vi "Master Setup Backup Scheduler.vi"(11 "Backup Path":path) -> ()   [LabVIEW 2017]
uses:
  Master Setup Backup Scheduler States.ctl
  <vilib>/Utility/config.llb/Read Key (Double).vi
  <vilib>/Utility/config.llb/Read Key (Boolean).vi
  <vilib>/Utility/config.llb/Read Key (U32).vi
  <vilib>/Utility/config.llb/Write Key (Double).vi
  <vilib>/Platform/browser.llb/Open URL in Default Browser (path).vi
  <vilib>/Utility/config.llb/Write Key (Boolean).vi
  <vilib>/Utility/config.llb/Write Key (U32).vi
  <vilib>/Utility/config.llb/NI_LVConfig.lvlib
panel:
  in  "Open Backup Directory":bool
  in  "Time Increment":enum32{"Days", "Weeks"}(ring)
  in  "Cancel":bool
  in  "Save":bool
  in  "Begin backup time":timestamp format="%<%b %d, %Y %I:%M %p>T"
  in  "Backup frequency":dbl
  out "Next scheduled backup":timestamp format="%<%b %d, %Y\n%I:%M %p>T"
  out "Last scheduled backup":timestamp format="%<%b %d, %Y\n%I:%M %p>T"
  in  "Auto Backup Enabled?":bool
  # "Back up the master setup files every"
  # "beginning on"
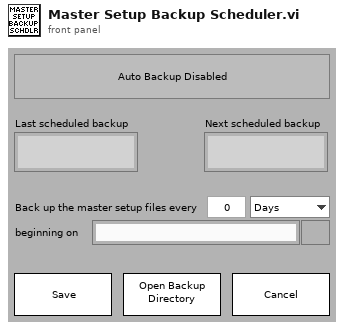
[diagram p1: front panel]
types:
  T1 = cluster{"Auto Backup Enabled?":bool, "Backup frequency":dbl, "Time Increment":enum32{"Days", "Weeks"}}
  T2 = typedef "Master Setup Backup Scheduler States.ctl" = enum16{"Initialize", "Enable/Disable controls", "Refresh controls", "Check for valid schdule", "Save", "Cancel", "Update", "Close", "Send backup command", "Update backup schedule", "Exit"}
  T3 = enum8{"Enabled", "Disabled", "Disabled and Grayed Out"}
  T4 = typedef "NI_LVConfig.lvlib/Config Data RefNum.ctl" = refnum<k1>
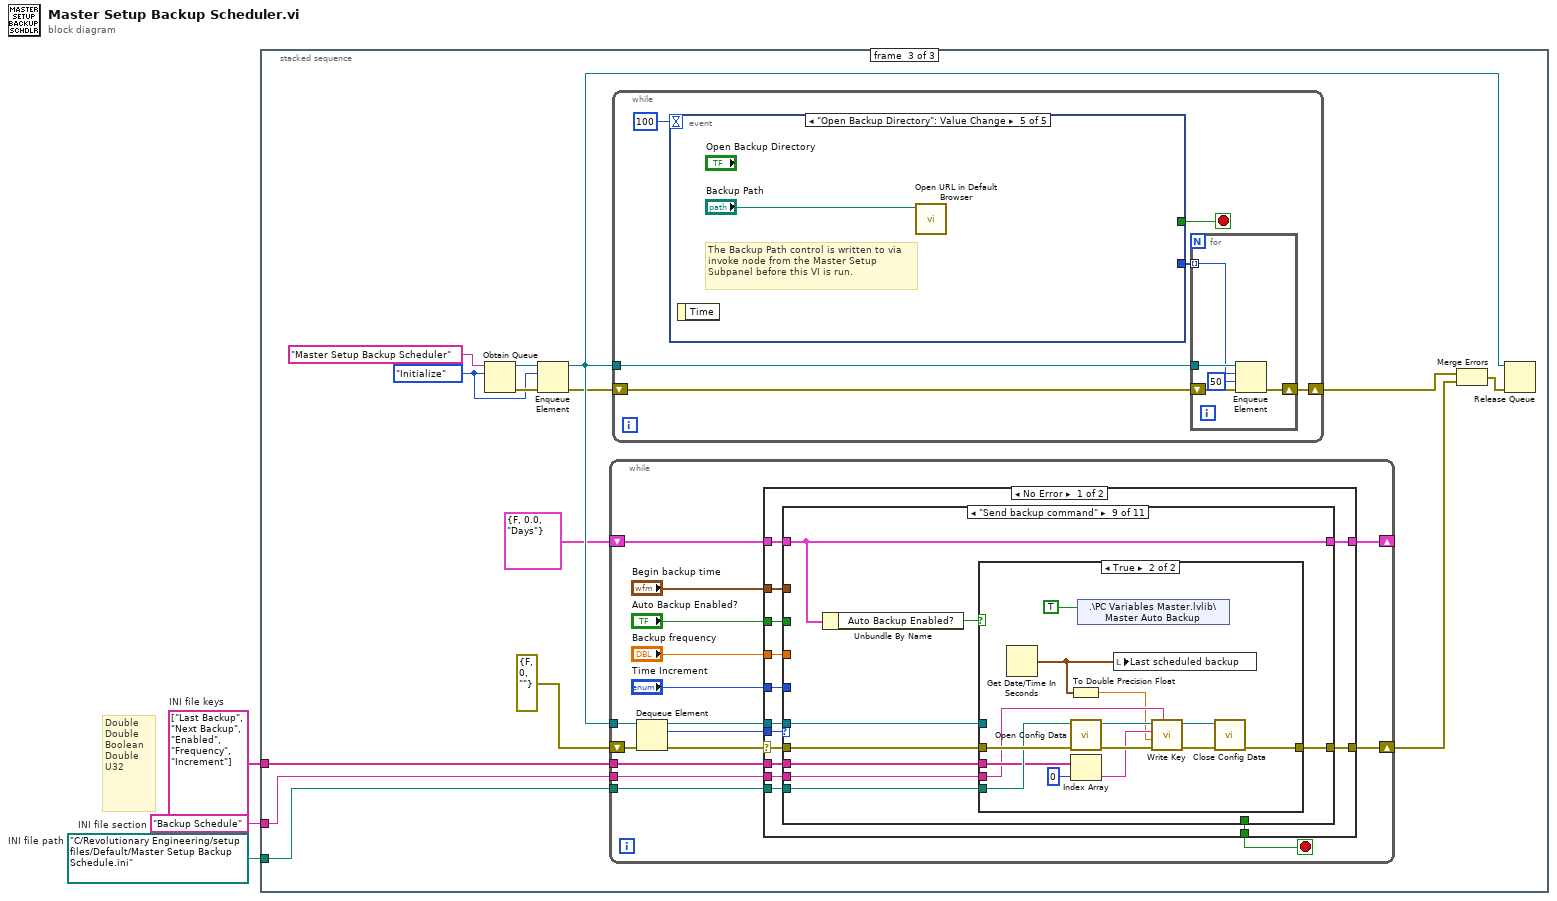
[diagram p0: block diagram]
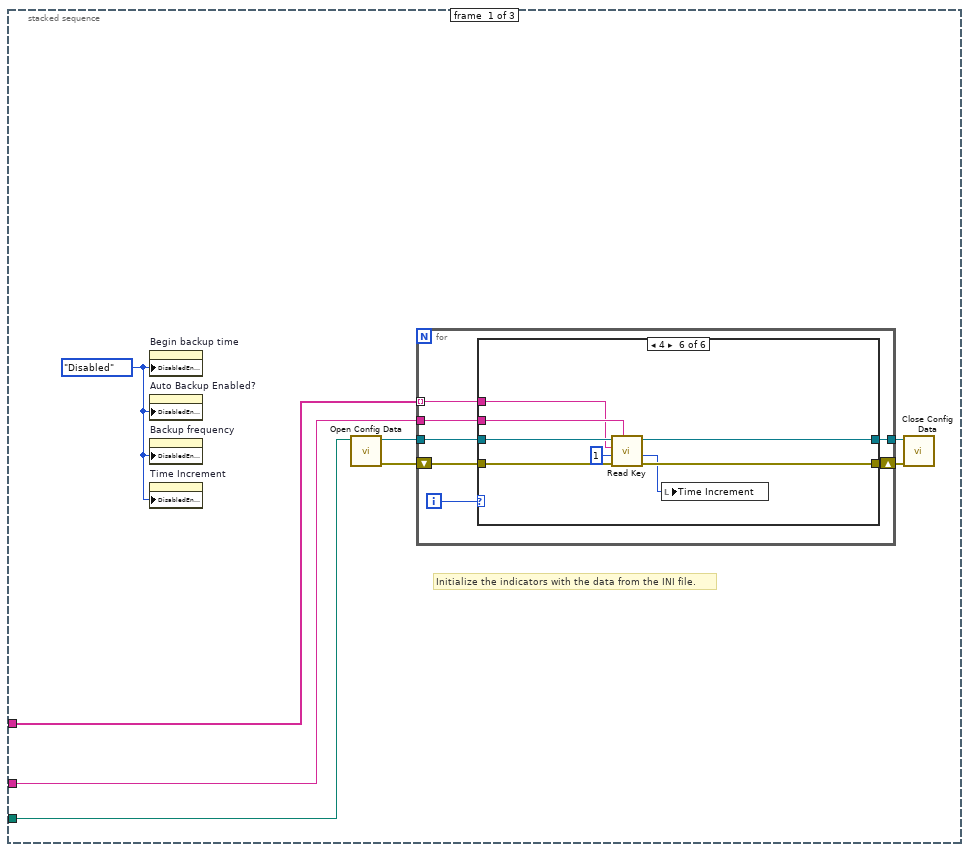
[diagram p2: hidden frame]
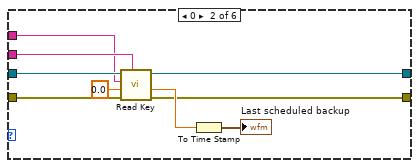
[diagram p4: hidden frame]
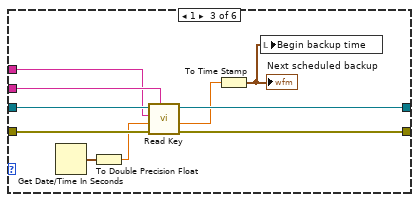
[diagram p5: hidden frame]
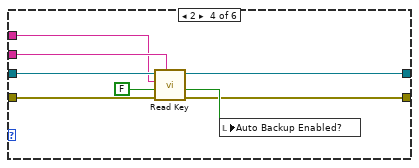
[diagram p6: hidden frame]
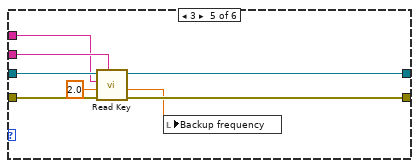
[diagram p7: hidden frame]
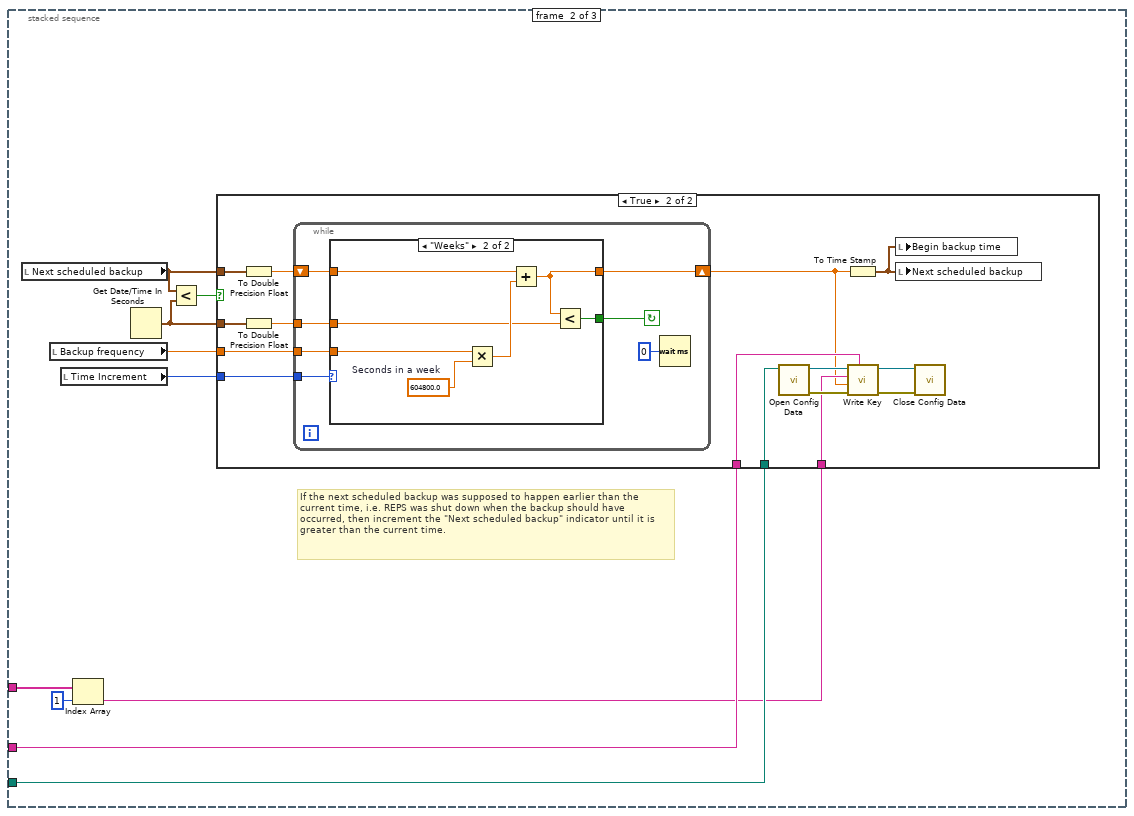
[diagram p8: hidden frame]
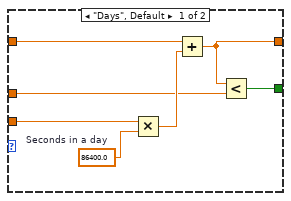
[diagram p10: hidden frame]
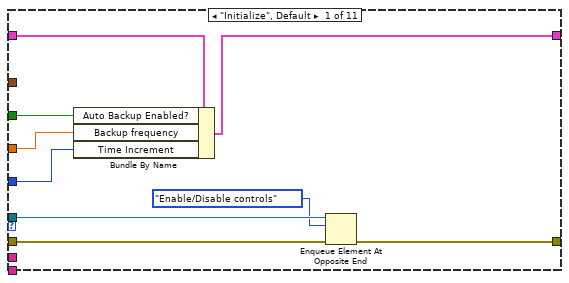
[diagram p11: hidden frame]
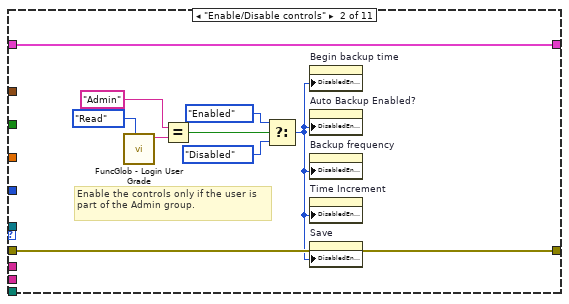
[diagram p12: hidden frame]
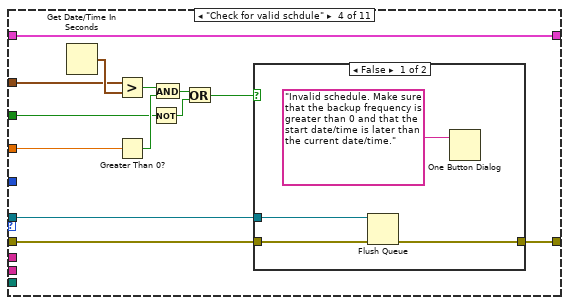
[diagram p14: hidden frame]
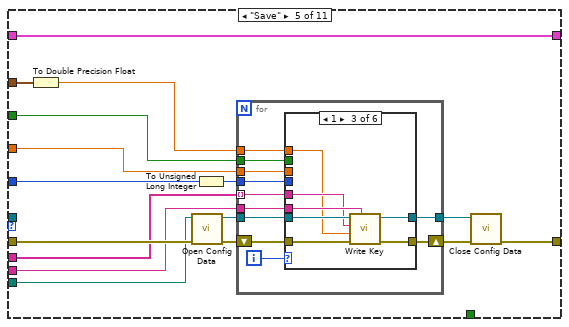
[diagram p16: hidden frame]
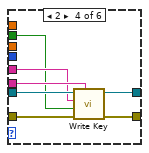
[diagram p19: hidden frame]
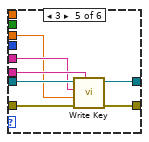
[diagram p20: hidden frame]
diagram:
  w1 = string[] ["Last Backup", "Next Backup", "Enabled", "Frequency", "Increment"]  # INI file keys
  w2 = "Backup Schedule"  # INI file section
  w3 = path "C:/Revolutionary Engineering/setup files/Default/Master Setup Backup Schedule.ini"  # INI file path
  # "Double\nDouble\nBoolean\nDouble\nU32"
  n1 = stacked-sequence {
    tunnel: w3 -> [w6 w68 w110]
    tunnel: w2 -> [w5 w67 w111]
    tunnel: w1 -> [w4 w66 w112]
    frame #0 {
      w7 = T3."Disabled" ("Disabled")
      # "Initialize the indicators with the data from the INI file."
      n2 = property on="Begin backup time" class="AbsTime (strict)"("DisabledEnum"=w7) -> ()  [unwired: 2 in, 2 out]
      n3 = property on="Auto Backup Enabled?" class="Bool (strict)"("DisabledEnum"=w7) -> ()  [unwired: 2 in, 2 out]
      n4 = property on="Backup frequency" class="DigNum (strict)"("DisabledEnum"=w7) -> ()  [unwired: 2 in, 2 out]
      n5 = property on="Time Increment" class="Enum (strict)"("DisabledEnum"=w7) -> ()  [unwired: 2 in, 2 out]
      n6 = call <vilib>:"Open Config Data.vi"("configuration file path"=w6) -> ("error out"=w10:errorcluster, "refnum"=w11:T4)  [unwired: 8 in, 1 out]
      n7 = for {
        tunnel: w11 -> [w17]
        tunnel: w5 -> [w14]
        tunnel: w4 -> [w15] mode=indexing
        shift-right: [w13] -> w9
        shift-left: w10 -> [w16]
        tunnel: [w12] -> w8
        i -> [w18]
        n8 = case shown="4" w18 {
          tunnel: w17 -> [w20 w29 w37 w47 w55 w63]
          tunnel: w16 -> [w19 w28 w39 w46 w54 w62]
          tunnel: w15 -> [_ w26 w34 w44 w52 w60]
          tunnel: w14 -> [_ w27 w35 w45 w53 w61]
          tunnel: [w19 w23 w38 w42 w50 w59] -> w13
          tunnel: [w20 w22 w36 w41 w51 w58] -> w12
          frame -1, Default {
          }
          frame 0 {
            n9 = call-poly <vilib>:"Read Key.vi"("section"=w27, "error in (no error)"=w28, "default value"=0.0, "key"=w26, "refnum"=w29) -> ("error out"=w23:errorcluster, "value"=w25:dbl, "refnum out"=w22:T4)  [unwired: 3 in, 1 out]
            n10 = To Time Stamp(1:w25) -> (0:→"Last scheduled backup":timestamp)
          }
          frame 1 {
            n11 = Get Date/Time In Seconds() -> (seconds since 1Jan1904=w32:timestamp)
            n12 = To Double Precision Float(number=w32) -> (double precision float=w31:dbl)
            n13 = call-poly <vilib>:"Read Key.vi"("section"=w35, "error in (no error)"=w39, "default value"=w31, "key"=w34, "refnum"=w37) -> ("error out"=w38:errorcluster, "value"=w33:dbl, "refnum out"=w36:T4)  [unwired: 3 in, 1 out]
            n14 = To Time Stamp(1:w33) -> (0:w30:timestamp)
            "Next scheduled backup" <- w30
            n15 = local write "Begin backup time"(w30) -> ()
          }
          frame 2 {
            n16 = call-poly <vilib>:"Read Key.vi"("section"=w45, "error in (no error)"=w46, "default value"=FALSE, "key"=w44, "refnum"=w47) -> ("error out"=w42:errorcluster, "value"=w43:bool, "refnum out"=w41:T4)  [unwired: 3 in, 1 out]
            n17 = local write "Auto Backup Enabled?"(w43) -> ()
          }
          frame 3 {
            n18 = call-poly <vilib>:"Read Key.vi"("section"=w53, "error in (no error)"=w54, "default value"=2.0, "key"=w52, "refnum"=w55) -> ("error out"=w50:errorcluster, "value"=w49:dbl, "refnum out"=w51:T4)  [unwired: 3 in, 1 out]
            n19 = local write "Backup frequency"(w49) -> ()
          }
          frame 4 {
            n20 = call-poly <vilib>:"Read Key.vi"("section"=w61, "error in (no error)"=w62, "default value"=u32 1, "key"=w60, "refnum"=w63) -> ("error out"=w59:errorcluster, "value"=w57:u32, "refnum out"=w58:T4)  [unwired: 3 in, 1 out]
            n21 = local write "Time Increment"(w57) -> ()
          }
        }
      }
      n22 = call <vilib>:"Close Config Data.vi"("error in (no error)"=w9, "refnum"=w8) -> ()  [unwired: 8 in, 2 out]
    }
    frame #1 {
      # "If the next scheduled backup was supposed to happen earlier than the current time, i.e. REPS was shut down when the backup should have occurred, then increment the \"Next scheduled backup\" indicator until it is greater than the current time."
      n23 = local read "Next scheduled backup"() -> (w70:timestamp)
      n24 = local read "Backup frequency"() -> (w72:dbl)
      n25 = local read "Time Increment"() -> (w71:enum32{"Days", "Weeks"})
      n26 = Index Array(array=w66, index=1) -> (element=w64:string)
      n27 = Get Date/Time In Seconds() -> (seconds since 1Jan1904=w69:timestamp)
      n28 = Less?(x=w70, y=w69) -> (x < y?=w73:bool)
      n29 = case shown="True" w73 {
        tunnel: w72 -> [_ w87]
        tunnel: w71 -> [_ w88]
        tunnel: w70 -> [_ w86]
        tunnel: w69 -> [_ w84]
        tunnel: w68 -> [_ w82]
        tunnel: w67 -> [_ w79]
        tunnel: w64 -> [_ w78]
        frame False {
        }
        frame True {
          n30 = To Double Precision Float(number=w86) -> (double precision float=w85:dbl)
          n31 = To Double Precision Float(number=w84) -> (double precision float=w83:dbl)
          n32 = while {
            tunnel: w88 -> [w95]
            tunnel: w87 -> [w94]
            tunnel: w83 -> [w92]
            shift-right: [w91] -> w77
            shift-left: w85 -> [w93]
            stop <- w90 continue-if-true
            n33 = case shown="\"Weeks\"" w95 {
              tunnel: w94 -> [w102 w105]
              tunnel: w93 -> [w99 w107]
              tunnel: w92 -> [w97 w106]
              tunnel: [w98 w103] -> w91
              tunnel: [w96 w104] -> w90
              frame "Days", Default {
                w101 = 86400.0  # Seconds in a day
                n34 = Multiply(x=w102, y=w101) -> (x*y=w100:dbl)
                n35 = Add(x=w99, y=w100) -> (x+y=w98:dbl)
                n36 = Less?(x=w98, y=w97) -> (x < y?=w96:bool)
              }
              frame "Weeks" {
                w109 = 604800.0  # Seconds in a week
                n37 = Multiply(x=w105, y=w109) -> (x*y=w108:dbl)
                n38 = Add(x=w107, y=w108) -> (x+y=w103:dbl)
                n39 = Less?(x=w103, y=w106) -> (x < y?=w104:bool)
              }
            }
            n40 = Wait (ms)(milliseconds to wait=u32 0) -> ()  [unwired: 1 out]
          }
          n41 = call <vilib>:"Open Config Data.vi"("configuration file path"=w82) -> ("error out"=w81:errorcluster, "refnum"=w80:T4)  [unwired: 8 in, 1 out]
          n42 = To Time Stamp(1:w77) -> (0:w74:timestamp)
          n43 = call-poly <vilib>:"Write Key.vi"("section"=w79, "error in (no error)"=w81, "value"=w77, "key"=w78, "refnum"=w80) -> ("error out"=w76:errorcluster, "refnum out"=w75:T4)  [unwired: 4 in, 1 out]
          n44 = local write "Begin backup time"(w74) -> ()
          n45 = local write "Next scheduled backup"(w74) -> ()
          n46 = call <vilib>:"Close Config Data.vi"("error in (no error)"=w76, "refnum"=w75) -> ()  [unwired: 8 in, 2 out]
        }
      }
    }
    frame #2 {
      w120 = Master_Setup_Backup_Scheduler_States."Initialize" ("Backup Scheduler States")
      n47 = Obtain Queue(name (unnamed)="Master Setup Backup Scheduler", element data type=w120) -> (queue out=w122:refnum<queue>, error out=w121:errorcluster)  [unwired: 3 in, 1 out]
      n48 = Enqueue Element(queue=w122, element=w120, error in (no error)=w121) -> (queue out=w118:refnum<queue>, error out=w114:errorcluster)  [unwired: 1 in, 1 out]
      n49 = while {
        tunnel: w118 -> [w139]
        shift-right: [w135] -> w116
        shift-left: errorcluster {"status"=FALSE, "code"=0, "source"=""} ("error out") -> [w138]
        shift-right: [w129] -> _
        shift-left: T1 {"Auto Backup Enabled?"=FALSE, "Backup frequency"=0.0, "Time Increment"=enum."Days"} -> [w133]
        tunnel: w112 -> [w127]
        tunnel: w111 -> [w126]
        tunnel: w110 -> [w125]
        stop <- w134 stop-if-true
        n50 = Dequeue Element(queue=w139, error in (no error)=w138) -> (queue out=w124:refnum<queue>, element=w137:T2, error out=w136:errorcluster)  [unwired: 1 in, 1 out]
        n51 = case shown="No Error" w136 {
          selector: w136 -> [w152 w319]
          tunnel: w137 -> [w153 _]
          tunnel: [w150 w318] -> w135
          tunnel: [w151 _] -> w134
          tunnel: w133 -> [w149 w317]
          tunnel: "Auto Backup Enabled?" -> [w148 _]
          tunnel: "Backup frequency" -> [w147 _]
          tunnel: "Time Increment" -> [w146 _]
          tunnel: [w145 w317] -> w129
          tunnel: "Begin backup time" -> [w144 _]
          tunnel: w127 -> [w143 _]
          tunnel: w126 -> [w142 _]
          tunnel: w125 -> [w141 _]
          tunnel: w124 -> [w140 _]
          frame No Error {
            n52 = case shown="\"Send backup command\"" w153 {
              tunnel: w152 -> [w157 w170 w172 w182 w207 w255 w257 w264 w272 w311 w315]
              tunnel: [_ _ _ _ _ _ _ _ _ _ TRUE] -> w151
              tunnel: [w156 w170 w172 w180 w198 w255 w257 w263 w268 w308 w315] -> w150
              tunnel: w149 -> [w162 w171 w173 w186 w192 w254 w262 w266 w274 w300 w314]
              tunnel: w148 -> [w161 _ _ w176 w197 _ w260 _ _ _ _]
              tunnel: w147 -> [w160 _ _ w183 w196 _ w259 _ _ _ _]
              tunnel: w146 -> [w159 _ _ _ w194 _ w258 _ _ _ _]
              tunnel: [w158 w171 w173 w186 w192 w254 w261 w266 w274 w300 w314] -> w145
              tunnel: w144 -> [_ _ _ w184 w193 _ w256 _ _ _ _]
              tunnel: w143 -> [_ _ _ _ w202 _ _ _ w271 w303 _]
              tunnel: w142 -> [_ _ _ _ w203 _ _ _ w270 w306 _]
              tunnel: w141 -> [_ _ _ _ w206 _ _ _ w269 w307 _]
              tunnel: w140 -> [w155 _ _ w181 _ _ _ _ w267 _ _]
              frame "Initialize", Default {
                n53 = Bundle By Name(cluster=w162, "Auto Backup Enabled?"=w161, "Backup frequency"=w160, "Time Increment"=w159) -> (w158:T1)
                n54 = Enqueue Element At Opposite End(queue=w155, element=Master_Setup_Backup_Scheduler_States."Enable/Disable controls" ("Backup Scheduler States"), error in (no error)=w157) -> (error out=w156:errorcluster)  [unwired: 1 in, 2 out]
              }
              frame "Enable/Disable controls" {
                # "Enable the controls only if the user is part of the Admin group."
                n55 = call "FuncGlob - Login User Grade.vi"("Action"=enum16{"Read", "Write"}."Read") -> ("Grade"=w167:string)  [unwired: 10 in]
                n56 = Equal?(x="Admin", y=w167) -> (x = y?=w166:bool)
                n57 = Select(t=T3."Enabled" ("Disabled"), s=w166, f=T3."Disabled" ("Disabled")) -> (s? t:f=w163:T3)
                n58 = property on="Begin backup time" class="AbsTime (strict)"("DisabledEnum"=w163) -> ()  [unwired: 2 in, 2 out]
                n59 = property on="Auto Backup Enabled?" class="Bool (strict)"("DisabledEnum"=w163) -> ()  [unwired: 2 in, 2 out]
                n60 = property on="Backup frequency" class="DigNum (strict)"("DisabledEnum"=w163) -> ()  [unwired: 2 in, 2 out]
                n61 = property on="Time Increment" class="Enum (strict)"("DisabledEnum"=w163) -> ()  [unwired: 2 in, 2 out]
                n62 = property on="Save" class="Bool"("DisabledEnum"=w163) -> ()  [unwired: 2 in, 2 out]
              }
              frame "Refresh controls" {
                # "The purpose of this case is to ensure that the most recent value of each of the controls is connected to the case sturcture. It is called when the user changes any of their values. No data processing should happen in this case."
              }
              frame "Check for valid schdule" {
                n63 = Get Date/Time In Seconds() -> (seconds since 1Jan1904=w185:timestamp)
                n64 = Greater?(x=w184, y=w185) -> (0:w179:bool)
                n65 = Greater Than 0?(x=w183) -> (x > 0?=w178:bool)
                n66 = Not(x=w176) -> (.not. x?=w175:bool)
                n67 = And(x=w179, y=w178) -> (x .and. y?=w177:bool)
                n68 = Or(x=w177, y=w175) -> (x .or. y?=w174:bool)
                n69 = case shown="False" w174 {
                  tunnel: w182 -> [w190 w191]
                  tunnel: w181 -> [w189 _]
                  tunnel: [w188 w191] -> w180
                  frame False {
                    n70 = Flush Queue(queue=w189, error in (no error)=w190) -> (error out=w188:errorcluster)  [unwired: 2 out]
                    n71 = One Button Dialog(message="Invalid schedule. Make sure that the backup frequency is greater than 0 and that the start date/time is later than the current date/time.") -> ()  [unwired: 1 in, 1 out]
                  }
                  frame True {
                  }
                }
              }
              frame "Save" {
                n72 = To Double Precision Float(number=w193) -> (double precision float=w201:dbl)
                n73 = call <vilib>:"Open Config Data.vi"("error in (no error)"=w207, "configuration file path"=w206) -> ("error out"=w204:errorcluster, "refnum"=w205:T4)  [unwired: 7 in, 1 out]
                n74 = To Unsigned Long Integer(number=w194) -> (unsigned 32bit integer=w195:u32)
                n75 = for {
                  tunnel: w205 -> [w218]
                  tunnel: w203 -> [w216]
                  shift-right: [w215] -> w200
                  shift-left: w204 -> [w217]
                  tunnel: w202 -> [w214] mode=indexing
                  tunnel: w195 -> [w212]
                  tunnel: w196 -> [w211]
                  tunnel: w197 -> [w210]
                  tunnel: w201 -> [w209]
                  tunnel: [w208] -> w199
                  i -> [w213]
                  n76 = case shown="1" w213 {
                    tunnel: w218 -> [w219 w221 w229 w236 w243 w250]
                    tunnel: w217 -> [w220 w222 w228 w235 w242 w249]
                    tunnel: w216 -> [_ _ w227 w234 w241 w248]
                    tunnel: [w220 w222 w226 w233 w240 w247] -> w215
                    tunnel: w214 -> [_ _ w225 w232 w239 w246]
                    tunnel: w212 -> [_ _ _ _ _ w245]
                    tunnel: w211 -> [_ _ _ _ w238 _]
                    tunnel: w210 -> [_ _ _ w231 _ _]
                    tunnel: w209 -> [_ _ w224 _ _ _]
                    tunnel: [w219 w221 w223 w230 w237 w244] -> w208
                    frame -1, Default {
                    }
                    frame 0 {
                      # "Don't write to the Last Backup key."
                    }
                    frame 1 {
                      n77 = call-poly <vilib>:"Write Key.vi"("section"=w227, "error in (no error)"=w228, "value"=w224, "key"=w225, "refnum"=w229) -> ("error out"=w226:errorcluster, "refnum out"=w223:T4)  [unwired: 4 in, 1 out]
                    }
                    frame 2 {
                      n78 = call-poly <vilib>:"Write Key.vi"("section"=w234, "error in (no error)"=w235, "value"=w231, "key"=w232, "refnum"=w236) -> ("error out"=w233:errorcluster, "refnum out"=w230:T4)  [unwired: 4 in, 1 out]
                    }
                    frame 3 {
                      n79 = call-poly <vilib>:"Write Key.vi"("section"=w241, "error in (no error)"=w242, "value"=w238, "key"=w239, "refnum"=w243) -> ("error out"=w240:errorcluster, "refnum out"=w237:T4)  [unwired: 4 in, 1 out]
                    }
                    frame 4 {
                      n80 = call-poly <vilib>:"Write Key.vi"("section"=w248, "error in (no error)"=w249, "value"=w245, "key"=w246, "refnum"=w250) -> ("error out"=w247:errorcluster, "refnum out"=w244:T4)  [unwired: 4 in, 1 out]
                    }
                  }
                }
                n81 = call <vilib>:"Close Config Data.vi"("error in (no error)"=w200, "refnum"=w199) -> ("error out"=w198:errorcluster)  [unwired: 8 in, 1 out]
              }
              frame "Cancel" {
                n82 = Unbundle By Name(w254) -> ("Auto Backup Enabled?"=w253:bool, "Backup frequency"=w251:dbl, "Time Increment"=w252:enum32{"Days", "Weeks"})
                n83 = local write "Auto Backup Enabled?"(w253) -> ()
                n84 = local write "Backup frequency"(w251) -> ()
                n85 = local write "Time Increment"(w252) -> ()
              }
              frame "Update" {
                n86 = local write "Begin backup time"(w256) -> ()
                n87 = local write "Next scheduled backup"(w256) -> ()
                n88 = Bundle By Name(cluster=w262, "Auto Backup Enabled?"=w260, "Backup frequency"=w259, "Time Increment"=w258) -> (w261:T1)
              }
              frame "Close" {
                n89 = control-ref of="This VI"() -> (w265:refnum<vi>)
                n90 = invoke class="VI" method="FP.Close"(reference=w265, error in=w264) -> (error out=w263:errorcluster)  [unwired: 1 in, 2 out]
              }
              frame "Send backup command" {
                n91 = Unbundle By Name(w274) -> ("Auto Backup Enabled?"=w273:bool)
                n92 = case shown="True" w273 {
                  tunnel: w272 -> [w277 w291]
                  tunnel: w271 -> [_ w287]
                  tunnel: w270 -> [_ w284]
                  tunnel: w269 -> [_ w290]
                  tunnel: [w276 w283] -> w268
                  tunnel: w267 -> [w275 _]
                  frame False {
                    n93 = Flush Queue(queue=w275, error in (no error)=w277) -> (error out=w276:errorcluster)  [unwired: 2 out]
                  }
                  frame True {
                    n94 = Get Date/Time In Seconds() -> (seconds since 1Jan1904=w279:timestamp)
                    n95 = To Double Precision Float(number=w279) -> (double precision float=w282:dbl)
                    n96 = call <vilib>:"Open Config Data.vi"("error in (no error)"=w291, "configuration file path"=w290) -> ("error out"=w288:errorcluster, "refnum"=w289:T4)  [unwired: 7 in, 1 out]
                    n97 = Index Array(array=w287, index=0) -> (element=w285:string)
                    n98 = shared-variable ".\\PC Variables Master.lvlib\\Master Auto Backup"(TRUE ("Master Auto Backup")) -> ()  [unwired: 1 in, 1 out]
                    n99 = local write "Last scheduled backup"(w279) -> ()
                    n100 = call-poly <vilib>:"Write Key.vi"("section"=w284, "error in (no error)"=w288, "value"=w282, "key"=w285, "refnum"=w289) -> ("error out"=w280:errorcluster, "refnum out"=w281:T4)  [unwired: 4 in, 1 out]
                    n101 = call <vilib>:"Close Config Data.vi"("error in (no error)"=w280, "refnum"=w281) -> ("error out"=w283:errorcluster)  [unwired: 8 in, 1 out]
                  }
                }
              }
              frame "Update backup schedule" {
                n102 = Unbundle By Name(w300) -> ("Time Increment"=w299:enum32{"Days", "Weeks"}, "Backup frequency"=w297:dbl)
                n103 = local read "Last scheduled backup"() -> (w293:timestamp)
                n104 = case shown="\"Days\", Default" w299 {
                  tunnel: [86400.0 604800.0] -> w298
                  frame "Days", Default {
                  }
                  frame "Weeks" {
                  }
                }
                n105 = To Double Precision Float(number=w293) -> (double precision float=w295:dbl)
                n106 = call <vilib>:"Open Config Data.vi"("error in (no error)"=w311, "configuration file path"=w307) -> ("error out"=w310:errorcluster, "refnum"=w305:T4)  [unwired: 7 in, 1 out]
                n107 = Index Array(array=w303, index=1) -> (element=w301:string)
                n108 = Multiply(x=w298, y=w297) -> (x*y=w296:dbl)
                n109 = Add(x=w295, y=w296) -> (x+y=w294:dbl)
                n110 = To Time Stamp(1:w294) -> (0:w292:timestamp)
                n111 = call-poly <vilib>:"Write Key.vi"("section"=w306, "error in (no error)"=w310, "value"=w294, "key"=w301, "refnum"=w305) -> ("error out"=w309:errorcluster, "refnum out"=w304:T4)  [unwired: 4 in, 1 out]
                n112 = local write "Begin backup time"(w292) -> ()
                n113 = local write "Next scheduled backup"(w292) -> ()
                n114 = call <vilib>:"Close Config Data.vi"("error in (no error)"=w309, "refnum"=w304) -> ("error out"=w308:errorcluster)  [unwired: 8 in, 1 out]
              }
              frame "Exit" {
              }
            }
          }
          frame Error {
            n115 = call <vilib>:"Clear Errors.vi"("error in (no error)"=w319) -> ("error out"=w318:errorcluster)  [unwired: 5 in, 1 out]
          }
        }
      }
      n116 = while {
        tunnel: w118 -> [w322]
        shift-right: [w320] -> w117
        shift-left: w114 -> [w321]
        stop <- w324 stop-if-true
        n117 = event shown="[4] \"Open Backup Directory\": Value Change" {
          selector: _ -> [_ _ _ _ _]
          dyn-events: _ -> [_ _ _ _ _]
          timeout: 100 -> [_ _ _ _ _]
          tunnel: [w331 _ _ _ _] -> w324
          tunnel: [w337 w349 w350 w351 _] -> w323
          event Timeout {
            w338 = T2[] [enum."Exit", enum."Enable/Disable controls", enum."Send backup command", enum."Update backup schedule"] items=["Initialize", "Enable/Disable controls", "Refresh controls", "Check for valid schdule", "Save", "Cancel", "Update", "Close", "Send backup command", "Update backup schedule", "Exit"]
            n118 = event-data() -> ()  [unwired: 1 in, 1 out]
            n119 = local read "Next scheduled backup"() -> (w344:timestamp)
            n120 = call "FuncGlob - Login User Grade.vi"("Action"=enum16{"Read", "Write"}."Read") -> ("Grade"=w334:string)  [unwired: 10 in]
            n121 = shared-variable ".\\PC Variables.lvlib\\Stop PC"() -> (w331:bool)  [unwired: 1 in, 1 out]
            n122 = feedback-in #1(w334) -> ()
            n123 = feedback #1() -> (w333:string)  [unwired: 1 in]
            n124 = Get Date/Time In Seconds() -> (seconds since 1Jan1904=w343:timestamp)
            n125 = Not Equal?(x=w334, y=w333) -> (x != y?=w332:bool)
            n126 = Greater Or Equal?(x=w343, y=w344) -> (x >= y?=w336:bool)
            n127 = Build Array(w331, w332, w336, w336) -> (w342:bool[])
            n128 = feedback-in #2(w342) -> ()
            n129 = feedback #2() -> (w341:bool[])  [unwired: 1 in]
            n130 = Greater?(x=w342, y=w341) -> (0:w339:bool[])
            n131 = Or Array Elements(Boolean array=w339) -> (logical OR=w340:bool)
            n132 = case shown="True" w340 {
              tunnel: w339 -> [_ w348]
              tunnel: w338 -> [_ w346]
              tunnel: [_ w345] -> w337
              frame False {
              }
              frame True {
                n133 = Not(x=w348) -> (.not. x?=w347:bool[])
                n134 = call "Delete items from array (U16).vi"("Items to delete"=w347, "Array"=w346) -> ("Array with items deleted"=w345:u16[])  [unwired: 9 in]
              }
            }
          }
          event "Save": Value Change {
            w349 = T2[] [enum."Check for valid schdule", enum."Save", enum."Update", enum."Close"] items=["Initialize", "Enable/Disable controls", "Refresh controls", "Check for valid schdule", "Save", "Cancel", "Update", "Close", "Send backup command", "Update backup schedule", "Exit"]
            n135 = event-data() -> ()  [unwired: 1 in, 1 out]
          }
          event "Cancel": Value Change; Panel Close {
            w350 = T2[] [enum."Cancel", enum."Close"] items=["Initialize", "Enable/Disable controls", "Refresh controls", "Check for valid schdule", "Save", "Cancel", "Update", "Close", "Send backup command", "Update backup schedule", "Exit"]
            n136 = event-data() -> ()  [unwired: 1 in, 1 out]
          }
          event "Begin backup time", "Auto Backup Enabled?", "Backup frequency", "Time Increment": Value Change {
            w351 = T2[] [enum."Refresh controls"] items=["Initialize", "Enable/Disable controls", "Refresh controls", "Check for valid schdule", "Save", "Cancel", "Update", "Close", "Send backup command", "Update backup schedule", "Exit"]
            n137 = event-data() -> ()  [unwired: 1 in, 1 out]
          }
          event "Open Backup Directory": Value Change {
            # "The Backup Path control is written to via invoke node from the Master Setup Subpanel before this VI is run."
            n138 = event-data() -> ()  [unwired: 1 in, 1 out]
            n139 = call-poly <vilib>:"Open URL in Default Browser.vi"("path"="Backup Path") -> ()  [unwired: 5 in, 2 out]
          }
        }
        n140 = for {
          tunnel: w323 -> [w329] mode=indexing
          tunnel: w322 -> [w330]
          shift-right: [w327] -> w320
          shift-left: w321 -> [w328]
          n141 = Enqueue Element(queue=w330, element=w329, timeout in ms (-1)=50, error in (no error)=w328) -> (error out=w327:errorcluster)  [unwired: 2 out]
        }
      }
      n142 = Merge Errors(w117, w116) -> (w115:errorcluster)
      n143 = Release Queue(queue=w118, error in (no error)=w115) -> ()  [unwired: 1 in, 3 out]
    }
  }
